vi "Action List.vi"() -> (0 "Action List":T1(array[cluster])=[{"Action Name"="Enable Motor", "JSON info"=[{"path"="Index", "data type"=enum."INT"}], "String Format"="%(Action Name) %(Index)"}, {"Action Name"="Disable Motor", "JSON info"=[{"path"="Index", "data type"=enum."INT"}], "String Format"="%(Action Name) %(Index)"}, {"Action Name"="Move Motor", "JSON info"=[{"path"="Index", "data type"=enum."INT"}, {"path"="Destination", "data type"=enum."DBL"}], "String Format"="%(Action Name) %(Index) to %(Destination)"}])   [LabVIEW 2016, in "Hardware.lvlib" / "Motions.lvlib" / "Motions.lvclass"]
uses:
  <userlib>/Common Components/Hardware/Abstract System/Motions/Motions/Motions.lvclass
panel:
  # "IMPORTANT!\nIf STRING is used, %s must be followed by a SPACE."
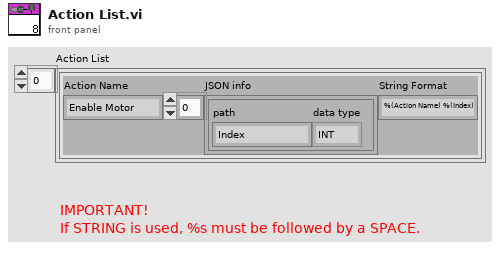
[diagram p1: front panel]
types:
  T1 = cluster{"Action Name":string, "JSON info":cluster{"path":string, "data type":enum16{"INT", "DBL", "BOOL", "String"}}[], "String Format":string}[]
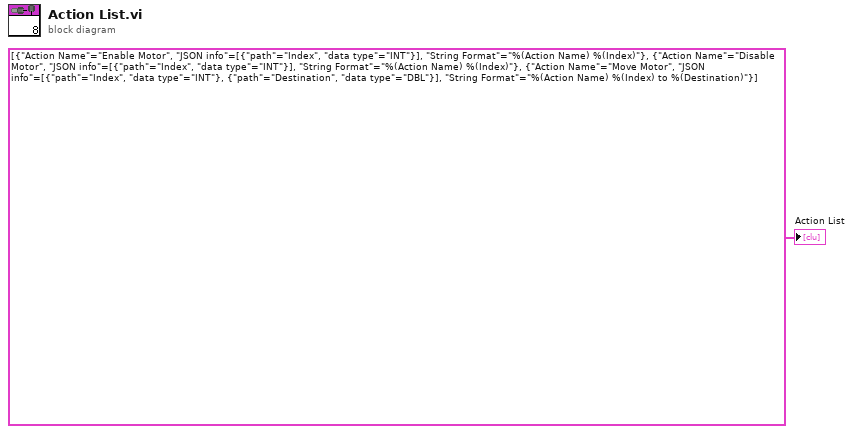
[diagram p0: block diagram]
diagram:
  "Action List" <- T1 [{"Action Name"="Enable Motor", "JSON info"=[{"path"="Index", "data type"=enum."INT"}], "String Format"="%(Action Name) %(Index)"}, {"Action Name"="Disable Motor", "JSON info"=[{"path"="Index", "data type"=enum."INT"}], "String Format"="%(Action Name) %(Index)"}, {"Action Name"="Move Motor", "JSON info"=[{"path"="Index", "data type"=enum."INT"}, {"path"="Destination", "data type"=enum."DBL"}], "String Format"="%(Action Name) %(Index) to %(Destination)"}]
